vi "DiodeTestAndCheck.vi"(0 "Diode Test Options":T1={"Temp.Tol"=0.1, "Max IDark"=[0.1, 1e-07], "Min ILight"=[0.15, 1e-06], "Min TEC \nCurrent"=0.2, "Max TEC \nCurrent"=1.0}, 1 "Stimulus_LED":refnum<vi>, 2 "DelayStr Ref":refnum<vi>, 3 "Diode Currents":refnum<vi>, 4 "TEC Faults Ref":refnum<vi>, 5 "CurrentTest":T2 {"Post-Log(s)" format="%#_13g"; "Pre-Log (s)" format="%#_13g"; "Duration (s)" format="%#_13g"}, 6 "Peltier_OnOffs":refnum<vi>, 11 "error in (no error)":errorcluster, 14 "TED Status":refnum<vi>) -> (15 "error out":errorcluster)   [LabVIEW 2025]
uses:
  controls/SingleTest.ctl
  controls/TestType.ctl
  controls/Diode Test Options.ctl
  <userlib>/_OpenG.lib/time/time.llb/openg_time.lvlib
panel:
  in  "CheckingTECCurrents":bool
  in  "CheckingTemperature":bool
  in  "CheckingConnections":bool
  out "TEC Faults":bool[](array[boolean])=[TRUE, TRUE]
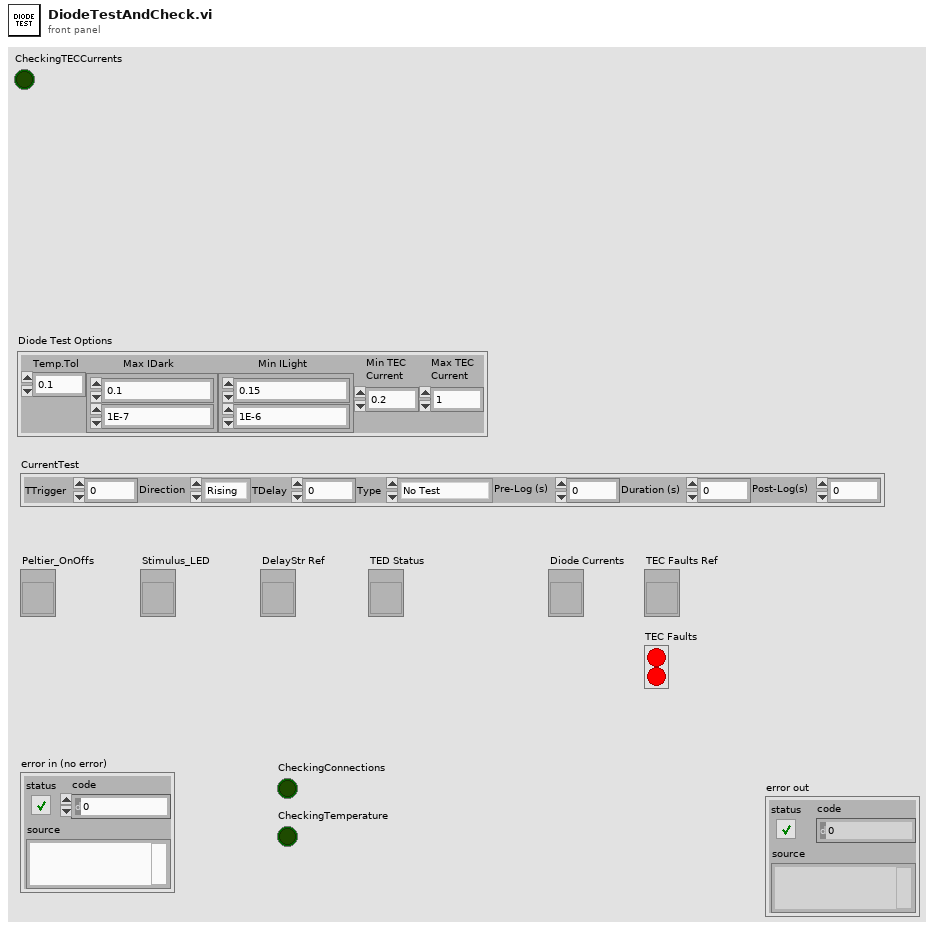
[diagram p1: front panel]
types:
  T1 = typedef "Diode Test Options.ctl" = cluster{"Temp.Tol":dbl, "Max IDark":dbl[], "Min ILight":dbl[], "Min TEC \nCurrent":dbl, "Max TEC \nCurrent":dbl}
  T2 = typedef "SingleTest.ctl" = cluster{"TTrigger":dbl, "Direction":enum16{"Rising", "Falling"}, "TDelay":dbl, "Type":T3, "Pre-Log (s)":dbl, "Duration (s)":dbl, "Post-Log(s)":dbl}
  T3 = typedef "TestType.ctl" = enum16{"No Test", "Heater Test", "Actuation Test", "Diode Test"}
  T4 = typedef "TED4015 Status.ctl" = cluster{"Output":bool, "SetPoint":dbl, "Temperature":dbl, "Current":dbl, "Voltage":dbl, "CableTrip":bool, "TransducerTrip":bool, "OverTemp":bool}
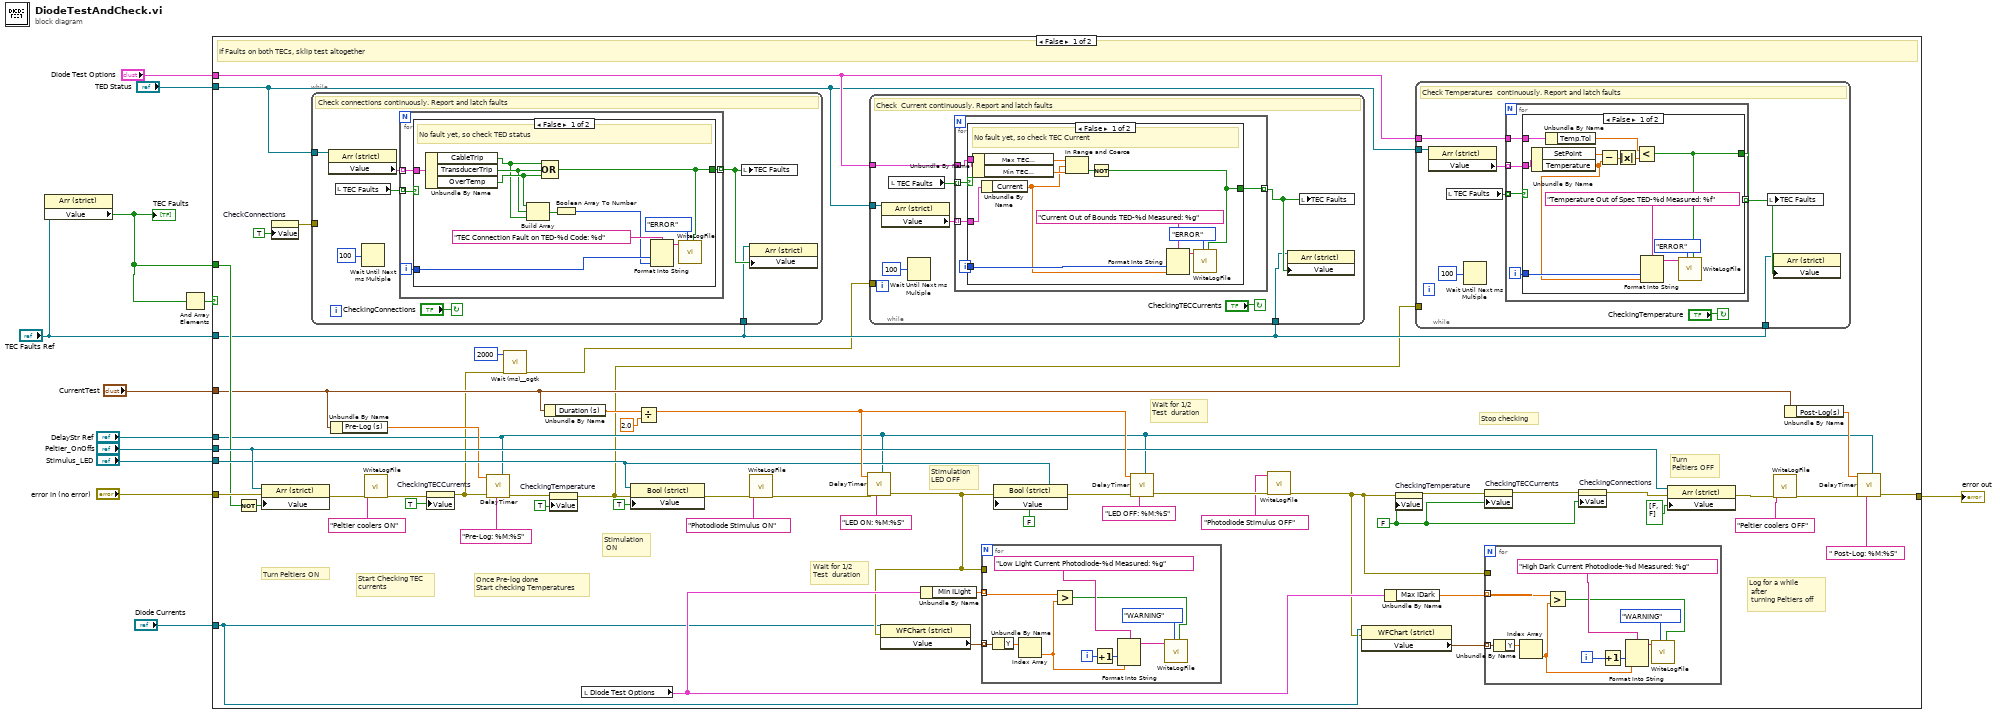
[diagram p0: block diagram]
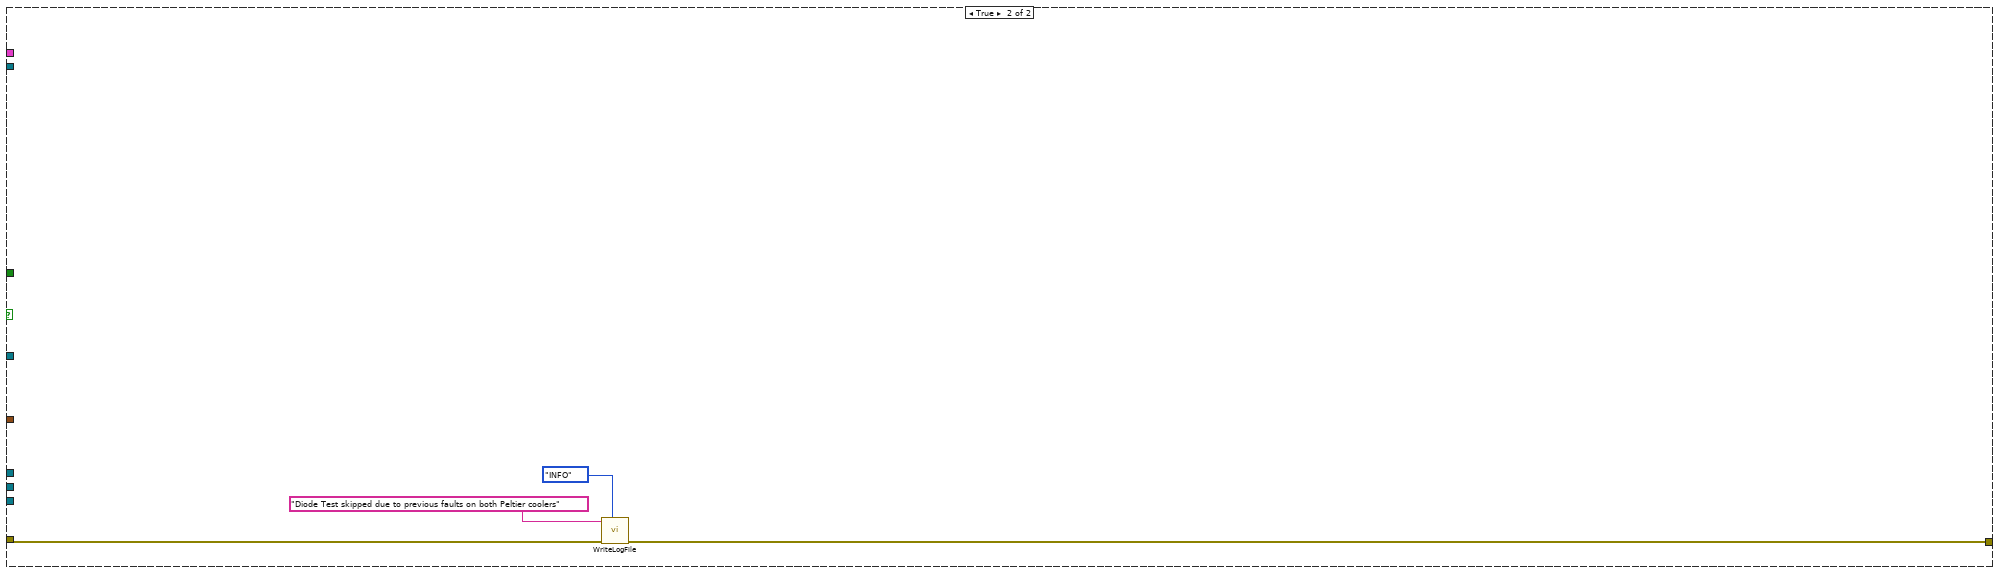
[diagram p5: hidden frame]
diagram:
  n1 = property class="Arr (strict)"(reference="TEC Faults Ref") -> ("Value"=w3:bool[])  [unwired: 1 in, 2 out]
  "TEC Faults" <- w3
  n2 = And Array Elements(Boolean array=w3) -> (logical AND=w7:bool)
  n3 = case shown="False" w7 {
    tunnel: "error in (no error)" -> [w54 w166]
    tunnel: "DelayStr Ref" -> [w47 _]
    tunnel: [w57 w165] -> w10
    tunnel: "Peltier_OnOffs" -> [w56 _]
    tunnel: "Stimulus_LED" -> [w55 _]
    tunnel: w3 -> [w49 _]
    tunnel: "TED Status" -> [w30 _]
    tunnel: "CurrentTest" -> [w45 _]
    tunnel: "Diode Currents" -> [w34 _]
    tunnel: "TEC Faults Ref" -> [w37 _]
    tunnel: "Diode Test Options" -> [w33 _]
    frame False {
      w39 = FALSE ("CheckingTemperature")
      # "Stop checking"
      # "Start Checking TEC\ncurrents"
      # "Once Pre-log done\nStart checking Temperatures"
      # "Stimulation\nLED OFF"
      # "Wait for 1/2 \nTest  duration"
      # "Stimulation\n ON"
      # "Log for a while\n after\n turning Peltiers off"
      # "Wait for 1/2 \nTest  duration"
      # "Turn \nPeltiers OFF"
      # "Turn Peltiers ON"
      # "If Faults on both TECs, sklip test altogether"
      n4 = Not(x=w49) -> (.not. x?=w53:bool[])
      n5 = property on="Property Node" class="Arr (strict)"(reference=w56, error in=w54, "Value"=w53) -> (error out=w20:errorcluster)  [unwired: 1 out]
      n6 = property on="CheckConnections" class="Bool (strict)"("Value"=TRUE ("CheckConnections")) -> (error out=w31:errorcluster)  [unwired: 2 in, 1 out]
      n7 = while {
        tunnel: w37 -> [w144]
        tunnel: w30 -> [w142]
        tunnel: w31 -> [_]
        stop <- "CheckingConnections" continue-if-true
        # "Check connections continuously. Report and latch faults"
        n8 = property class="Arr (strict)"(reference=w142) -> ("Value"=w143:T4[])  [unwired: 1 in, 2 out]
        n9 = local read "TEC Faults"() -> (w141:bool[])
        n10 = Wait Until Next ms Multiple(millisecond multiple=u32 100) -> ()  [unwired: 1 out]
        n11 = for {
          tunnel: w143 -> [w150] mode=indexing
          tunnel: w141 -> [w147] mode=indexing
          tunnel: [w148] -> w145 mode=indexing
          i -> [w149]
          n12 = case shown="False" w147 {
            selector: w147 -> [_ w162]
            tunnel: w150 -> [w161 _]
            tunnel: w149 -> [w159 _]
            tunnel: [w156 w162] -> w148
            frame False {
              # "No fault yet, so check TED status"
              n13 = Unbundle By Name(w161) -> ("CableTrip"=w153:bool, "TransducerTrip"=w154:bool, "OverTemp"=w155:bool)
              n14 = Build Array(w155, w154, w153) -> (w152:bool[])
              n15 = Compound Arithmetic op=OR(w153, w154, w155) -> (w156:bool)
              n16 = Boolean Array To Number(Boolean array=w152) -> (number=w151:u32)
              n17 = Format Into String(format string="TEC Connection Fault on TED-%d Code: %d", w159, w151) -> (resulting string=w158:string)  [unwired: 2 in, 1 out]
              n18 = call "WriteLogFile.vi"("Write?"=w156, "Type"=enum16{"INFO", "WARNING", "ERROR"}."ERROR", "Message"=w158) -> ()  [unwired: 8 in, 1 out]
            }
            frame True {
              # "Fault detected, so latch and don't check again on this channel"
            }
          }
        }
        n19 = local write "TEC Faults"(w145) -> ()
        n20 = property class="Arr (strict)"(reference=w144, "Value"=w145) -> ()  [unwired: 1 in, 2 out]
      }
      n21 = Unbundle By Name(w45) -> ("Pre-Log (s)"=w52:dbl)
      n22 = call "WriteLogFile.vi"("error in (no error)"=w20, "Message"="Peltier coolers ON") -> ("error out"=w21:errorcluster)  [unwired: 9 in]
      n23 = property on="CheckingTECCurrents" class="Bool (strict)"(error in=w21, "Value"=TRUE ("CheckingTECCurrents")) -> (error out=w15:errorcluster)  [unwired: 1 in, 1 out]
      n24 = call "DelayTimer.vi"("Formatted \nTime Ref"=w47, "FormatString"="Pre-Log: %M:%S", "error in (no error)"=w15, "Delay(s)"=w52) -> ("error out"=w51:errorcluster)  [unwired: 7 in]
      n25 = call <userlib>:"Wait (ms)__ogtk.vi"("error in (no error)"=w15, "milliseconds to wait"=u32 2000) -> ("error out"=w14:errorcluster)  [unwired: 8 in, 1 out]
      n26 = Unbundle By Name(w45) -> ("Duration (s)"=w44:dbl)
      n27 = property on="CheckingTemperature" class="Bool (strict)"(error in=w51, "Value"=TRUE ("CheckingTemperature")) -> (error out=w28:errorcluster)  [unwired: 1 in, 1 out]
      n28 = local read "Diode Test Options"() -> (w38:T1)
      n29 = property on="Property Node" class="Bool (strict)"(reference=w55, error in=w28, "Value"=TRUE ("LED_Stimulate")) -> (error out=w26:errorcluster)  [unwired: 1 out]
      n30 = Divide(x=w44, y=2.0) -> (x/y=w67:dbl)
      n31 = call "WriteLogFile.vi"("error in (no error)"=w26, "Message"="Photodiode Stimulus ON") -> ("error out"=w27:errorcluster)  [unwired: 9 in]
      n32 = call "DelayTimer.vi"("Formatted \nTime Ref"=w47, "FormatString"="LED ON: %M:%S", "error in (no error)"=w27, "Delay(s)"=w67) -> ("error out"=w36:errorcluster)  [unwired: 7 in]
      n33 = while {
        tunnel: w33 -> [w96]
        tunnel: w37 -> [w93]
        tunnel: w30 -> [w91]
        tunnel: w14 -> [_]
        stop <- "CheckingTECCurrents" continue-if-true
        # "Check  Current continuously. Report and latch faults"
        n34 = property class="Arr (strict)"(reference=w91) -> ("Value"=w92:T4[])  [unwired: 1 in, 2 out]
        n35 = local read "TEC Faults"() -> (w90:bool[])
        n36 = Wait Until Next ms Multiple(millisecond multiple=u32 100) -> ()  [unwired: 1 out]
        n37 = for {
          tunnel: w92 -> [w101] mode=indexing
          tunnel: w96 -> [w100]
          tunnel: w90 -> [w97] mode=indexing
          tunnel: [w98] -> w94 mode=indexing
          i -> [w99]
          n38 = case shown="False" w97 {
            selector: w97 -> [_ w113]
            tunnel: w101 -> [w112 _]
            tunnel: w100 -> [w110 _]
            tunnel: w99 -> [w106 _]
            tunnel: [w103 w113] -> w98
            frame False {
              # "No fault yet, so check TEC Current"
              n39 = Unbundle By Name(w110) -> ("Max TEC \nCurrent"=w108:dbl, "Min TEC \nCurrent"=w109:dbl)
              n40 = Unbundle By Name(w112) -> ("Current"=w102:dbl)
              n41 = In Range and Coerce(upper limit=w108, x=w102, lower limit=w109) -> (In Range?=w111:bool)  [unwired: 1 out]
              n42 = Not(x=w111) -> (.not. x?=w103:bool)
              n43 = Format Into String(format string="Current Out of Bounds TED-%d Measured: %g", w106, w102) -> (resulting string=w105:string)  [unwired: 2 in, 1 out]
              n44 = call "WriteLogFile.vi"("Write?"=w103, "Type"=enum16{"INFO", "WARNING", "ERROR"}."ERROR", "Message"=w105) -> ()  [unwired: 8 in, 1 out]
            }
            frame True {
            }
          }
        }
        n45 = property class="Arr (strict)"(reference=w93, "Value"=w94) -> ()  [unwired: 1 in, 2 out]
        n46 = local write "TEC Faults"(w94) -> ()
      }
      n47 = property class="WFChart (strict)"(reference=w34, error in=w36) -> ("Value"=w43:waveform(dbl)[])  [unwired: 2 out]
      n48 = Unbundle By Name(w38) -> ("Min ILight"=w46:dbl[])
      n49 = for {
        tunnel: w46 -> [w84] mode=indexing
        tunnel: w43 -> [w86] mode=indexing
        tunnel: w36 -> [_]
        i -> [w88]
        n50 = Unbundle By Name(w86) -> ("Y"=w85:dbl[])
        n51 = Index Array(array=w85) -> (element=w79:dbl)  [unwired: 1 in]
        n52 = Greater?(x=w84, y=w79) -> (0:w80:bool)
        n53 = Increment(x=w88) -> (x+1=w81:i32)
        n54 = Format Into String(format string="Low Light Current Photodiode-%d Measured: %g", w81, w79) -> (resulting string=w83:string)  [unwired: 2 in, 1 out]
        n55 = call "WriteLogFile.vi"("Write?"=w80, "Type"=enum16{"INFO", "WARNING", "ERROR"}."WARNING", "Message"=w83) -> ()  [unwired: 8 in, 1 out]
      }
      n56 = property on="Property Node" class="Bool (strict)"(reference=w55, error in=w36, "Value"=FALSE ("LED_Stimulate")) -> (error out=w66:errorcluster)  [unwired: 1 out]
      n57 = call "DelayTimer.vi"("Formatted \nTime Ref"=w47, "FormatString"="LED OFF: %M:%S", "error in (no error)"=w66, "Delay(s)"=w67) -> ("error out"=w23:errorcluster)  [unwired: 7 in]
      n58 = call "WriteLogFile.vi"("error in (no error)"=w23, "Message"="Photodiode Stimulus OFF") -> ("error out"=w24:errorcluster)  [unwired: 9 in]
      n59 = property class="WFChart (strict)"(reference=w34, error in=w24) -> ("Value"=w35:waveform(dbl)[])  [unwired: 2 out]
      n60 = Unbundle By Name(w38) -> ("Max IDark"=w42:dbl[])
      n61 = property on="CheckingTemperature" class="Bool (strict)"(error in=w24, "Value"=w39) -> (error out=w29:errorcluster)  [unwired: 1 in, 1 out]
      n62 = while {
        tunnel: w33 -> [w121]
        tunnel: w37 -> [w118]
        tunnel: w30 -> [w116]
        tunnel: w28 -> [_]
        stop <- "CheckingTemperature" continue-if-true
        # "Check Temperatures  continuously. Report and latch faults"
        n63 = property class="Arr (strict)"(reference=w116) -> ("Value"=w117:T4[])  [unwired: 1 in, 2 out]
        n64 = local read "TEC Faults"() -> (w115:bool[])
        n65 = Wait Until Next ms Multiple(millisecond multiple=u32 100) -> ()  [unwired: 1 out]
        n66 = for {
          tunnel: w117 -> [w126] mode=indexing
          tunnel: w121 -> [w125]
          tunnel: w115 -> [w122] mode=indexing
          tunnel: [w124] -> w119 mode=indexing
          i -> [w123]
          n67 = case shown="False" w122 {
            selector: w122 -> [_ w139]
            tunnel: w126 -> [w138 _]
            tunnel: w125 -> [w135 _]
            tunnel: [w128 w139] -> w124
            tunnel: w123 -> [w131 _]
            frame False {
              n68 = Unbundle By Name(w138) -> ("SetPoint"=w133:dbl, "Temperature"=w127:dbl)
              n69 = Unbundle By Name(w135) -> ("Temp.Tol"=w134:dbl)
              n70 = Subtract(x=w133, y=w127) -> (x-y=w137:dbl)
              n71 = Absolute Value(x=w137) -> (abs(x)=w136:dbl)
              n72 = Less?(x=w134, y=w136) -> (x < y?=w128:bool)
              n73 = Format Into String(format string="Temperature Out of Spec TED-%d Measured: %f", w131, w127) -> (resulting string=w130:string)  [unwired: 2 in, 1 out]
              n74 = call "WriteLogFile.vi"("Write?"=w128, "Type"=enum16{"INFO", "WARNING", "ERROR"}."ERROR", "Message"=w130) -> ()  [unwired: 8 in, 1 out]
            }
            frame True {
            }
          }
        }
        n75 = local write "TEC Faults"(w119) -> ()
        n76 = property class="Arr (strict)"(reference=w118, "Value"=w119) -> ()  [unwired: 1 in, 2 out]
      }
      n77 = for {
        tunnel: w42 -> [w74] mode=indexing
        tunnel: w35 -> [w76] mode=indexing
        tunnel: w24 -> [_]
        i -> [w78]
        n78 = Unbundle By Name(w76) -> ("Y"=w75:dbl[])
        n79 = Index Array(array=w75) -> (element=w69:dbl)  [unwired: 1 in]
        n80 = Greater?(x=w74, y=w69) -> (0:w70:bool)
        n81 = Increment(x=w78) -> (x+1=w71:i32)
        n82 = Format Into String(format string="High Dark Current Photodiode-%d Measured: %g", w71, w69) -> (resulting string=w73:string)  [unwired: 2 in, 1 out]
        n83 = call "WriteLogFile.vi"("Write?"=w70, "Type"=enum16{"INFO", "WARNING", "ERROR"}."WARNING", "Message"=w73) -> ()  [unwired: 8 in, 1 out]
      }
      n84 = property on="CheckingTECCurrents" class="Bool (strict)"(error in=w29, "Value"=w39) -> (error out=w41:errorcluster)  [unwired: 1 in, 1 out]
      n85 = property on="CheckingConnections" class="Bool (strict)"(error in=w41, "Value"=w39) -> (error out=w40:errorcluster)  [unwired: 1 in, 1 out]
      n86 = property on="Property Node" class="Arr (strict)"(reference=w56, error in=w40, "Value"=bool[] [FALSE, FALSE]) -> (error out=w17:errorcluster)  [unwired: 1 out]
      n87 = call "WriteLogFile.vi"("error in (no error)"=w17, "Message"="Peltier coolers OFF") -> ("error out"=w16:errorcluster)  [unwired: 9 in]
      n88 = Unbundle By Name(w45) -> ("Post-Log(s)"=w62:dbl)
      n89 = call "DelayTimer.vi"("Formatted \nTime Ref"=w47, "FormatString"=" Post-Log: %M:%S", "error in (no error)"=w16, "Delay(s)"=w62) -> ("error out"=w57:errorcluster)  [unwired: 7 in]
    }
    frame True {
      n90 = call "WriteLogFile.vi"("Type"=enum16{"INFO", "WARNING", "ERROR"}."INFO", "error in (no error)"=w166, "Message"="Diode Test skipped due to previous faults on both Peltier coolers") -> ("error out"=w165:errorcluster)  [unwired: 8 in]
    }
  }
  "error out" <- w10
